vi "RTP_RTSP - Get Parameter (I32).vi"(5 "Name":string, 8 "error in":errorcluster, 9 "Data":string) -> (0 "error out":errorcluster, 1 "Parameter (I32)":i32)   [LabVIEW 2014]
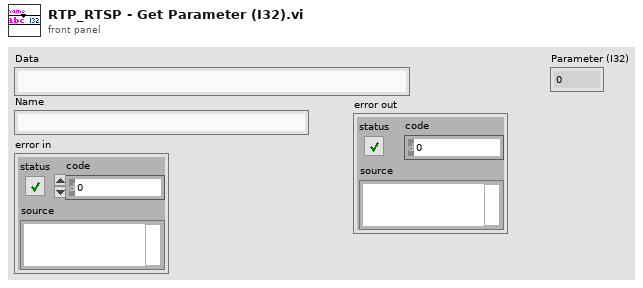
[diagram p1: front panel]
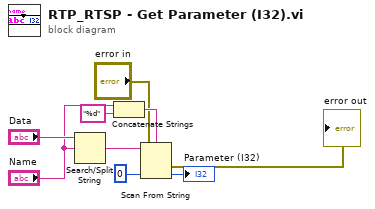
[diagram p0: block diagram]
diagram:
  n1 = Search/Split String(string="Data", search string/char (-)="Name") -> (match + rest of string=w9:string)  [unwired: 1 in, 2 out]
  n2 = Concatenate Strings("Name", "%d" ("format string")) -> (w7:string)
  n3 = Scan From String(format string=w7, input string=w9, error in="error in", default 1=0) -> (error out=→"error out":errorcluster, output 1=→"Parameter (I32)":i32)  [unwired: 1 in, 2 out]
